vi "Update PPL Build Specs.vi"(8 "error in (no error)":errorcluster, 11 "Pre-Build Properties":T1) -> (0 "error out":errorcluster, 3 "Pre-Build Properties dup":T1)   [LabVIEW 2020]
uses:
  pre-build properties -- cluster.ctl
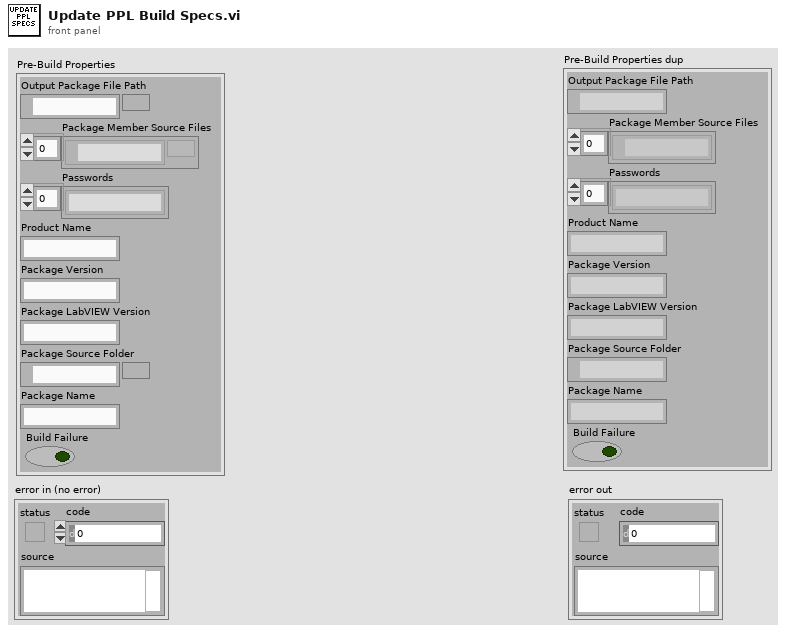
[diagram p1: front panel]
types:
  T1 = typedef "pre-build properties -- cluster.ctl" = cluster{"Output Package File Path":path, "Package Member Source Files":path[], "Passwords":string[], "Product Name":string, "Package Version":string, "Package LabVIEW Version":string, "Package Source Folder":path, "Package Name":string, "Build Failure":bool}
  T2 = enum16{"open", "replace", "create", "open or create", "replace or create", "replace or create with confirmation"}
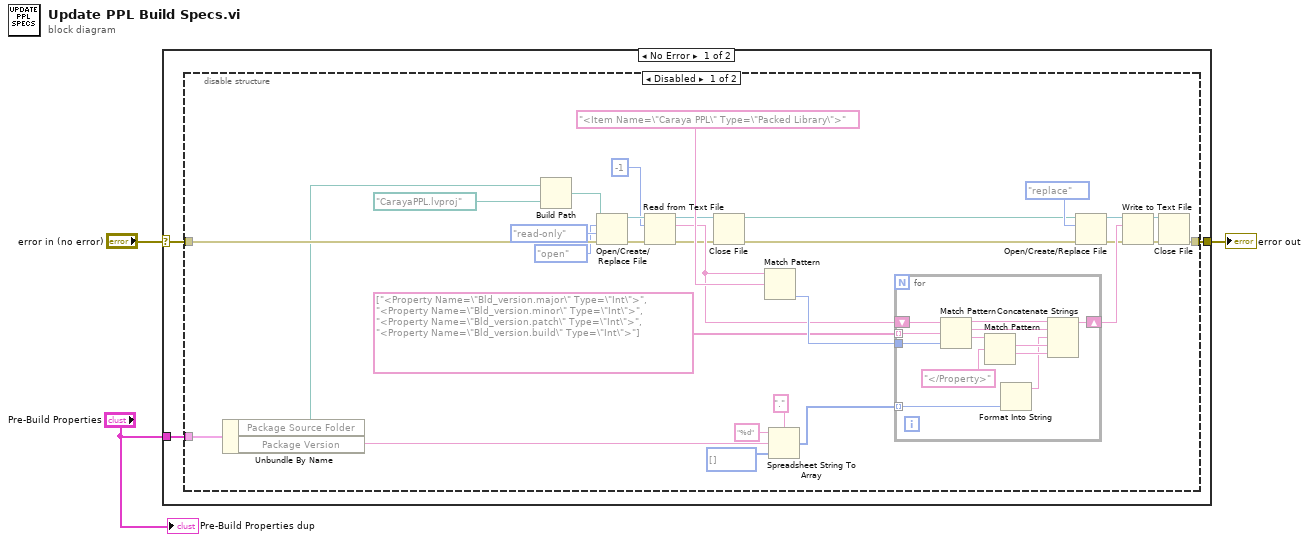
[diagram p0: block diagram]
diagram:
  n1 = case shown="No Error" "error in (no error)" {
    selector: "error in (no error)" -> [w5 w50]
    tunnel: [w4 w50] -> w3
    tunnel: "Pre-Build Properties" -> [w6 _]
    frame No Error {
      n2 = disable-structure shown="Disabled" {
        disable-tunnel: w6 -> [w35 _]
        disable-tunnel: w5 -> [w33 w49]
        disable-tunnel: [w26 w49] -> w4
        frame Disabled {
          n3 = Unbundle By Name(w35) -> ("Package Source Folder"=w7:path, "Package Version"=w8:string)
          n4 = Build Path(base path=w7, name or relative path=path "CarayaPPL.lvproj" ("base path")) -> (appended path=w30:path)
          n5 = Open/Create/Replace File(file path (use dialog)=w30, error in=w33, operation (0:open)=T2."open", access (0:read/write)=enum16{"read/write", "read-only", "write-only"}."read-only") -> (refnum out=w31:refnum<file>, error out=w32:errorcluster)  [unwired: 2 in, 1 out]
          n6 = Read from Text File(file (use dialog)=w31, count=-1, error in=w32) -> (refnum out=w20:refnum<file>, text=w21:string, error out=w19:errorcluster)  [unwired: 1 in, 1 out]
          n7 = Close File(refnum=w20, error in=w19) -> (path=w15:path, error out=w18:errorcluster)
          n8 = Match Pattern(string=w21, regular expression="<Item Name=\"Caraya PPL\" Type=\"Packed Library\">") -> (offset past match=w23:i32)  [unwired: 1 in, 3 out]
          n9 = Spreadsheet String To Array(delimiter (Tab)=".", format string="%d", spreadsheet string=w8, array type (2D Dbl)=u16[] []) -> (array=w9:u16[])
          n10 = for {
            tunnel: string[] ["<Property Name=\"Bld_version.major\" Type=\"Int\">", "<Property Name=\"Bld_version.minor\" Type=\"Int\">", "<Property Name=\"Bld_version.patch\" Type=\"Int\">", "<Property Name=\"Bld_version.build\" Type=\"Int\">"] -> [w48] mode=indexing
            tunnel: w23 -> [w41]
            shift-right: [w42] -> w34
            shift-left: w21 -> [w40]
            tunnel: w9 -> [w37] mode=indexing
            n11 = Match Pattern(string=w40, regular expression=w48, offset (0)=w41) -> (before substring=w46:string, match substring=w45:string, after substring=w47:string)  [unwired: 1 out]
            n12 = Match Pattern(string=w47, regular expression="</Property>") -> (match substring=w44:string, after substring=w43:string)  [unwired: 1 in, 2 out]
            n13 = Format Into String(w37) -> (resulting string=w38:string)  [unwired: 3 in, 1 out]
            n14 = Concatenate Strings(w46, w45, w38, w44, w43) -> (w42:string)
          }
          n15 = Open/Create/Replace File(file path (use dialog)=w15, error in=w18, operation (0:open)=T2."replace") -> (refnum out=w14:refnum<file>, error out=w17:errorcluster)  [unwired: 3 in, 1 out]
          n16 = Write to Text File(file (use dialog)=w14, text=w34, error in=w17) -> (refnum out=w25:refnum<file>, error out=w27:errorcluster)  [unwired: 1 in, 1 out]
          n17 = Close File(refnum=w25, error in=w27) -> (error out=w26:errorcluster)  [unwired: 1 out]
        }
        frame Enabled {
        }
      }
    }
    frame Error {
    }
  }
  "error out" <- w3
  "Pre-Build Properties dup" <- "Pre-Build Properties"
